vi "setParameters.vi"(10 "Parameters":T1, 11 "AbortRaiseM1M3Command in":refnum<class "AbortRaiseM1M3Command.lvclass">) -> (3 "AbortRaiseM1M3Command out":refnum<class "AbortRaiseM1M3Command.lvclass">)   [LabVIEW 2016, in "AbortRaiseM1M3Command.lvclass"]
uses:
  AbortRaiseM1M3Command.lvclass
  DataTypes/Topics/CommandAbortRaiseM1M3.ctl
  DataTypes/Topics/Parts/CommandId.ctl
  AbortRaiseM1M3Command.lvclass/AbortRaiseM1M3Command.ctl
  DataTypes/Topics/M1M3SupportTopics.lvlib
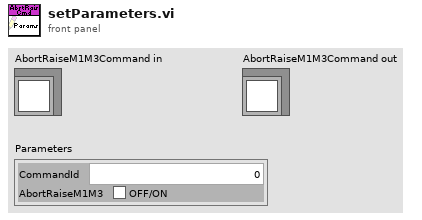
[diagram p1: front panel]
types:
  T1 = typedef "M1M3SupportTopics.lvlib/CommandAbortRaiseM1M3.ctl" = cluster{"CommandId":T2, "AbortRaiseM1M3":bool}
  T2 = typedef "M1M3SupportTopics.lvlib/CommandId.ctl" = i32
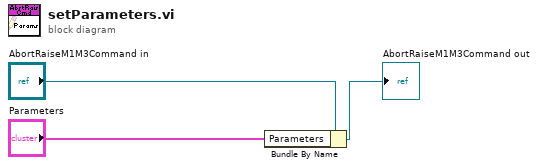
[diagram p0: block diagram]
diagram:
  n1 = Bundle By Name(cluster="AbortRaiseM1M3Command in", "Parameters"="Parameters") -> (→"AbortRaiseM1M3Command out":refnum<class "AbortRaiseM1M3Command.lvclass">)
